vi "MosbusResponseSubVI.vi"(0 "Read String":string) -> (1 "Function Code":i32, 2 "Byte Count":i32, 3 "Data":dbl)   [LabVIEW 2016]
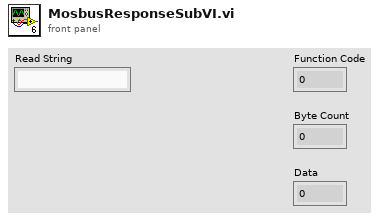
[diagram p1: front panel]
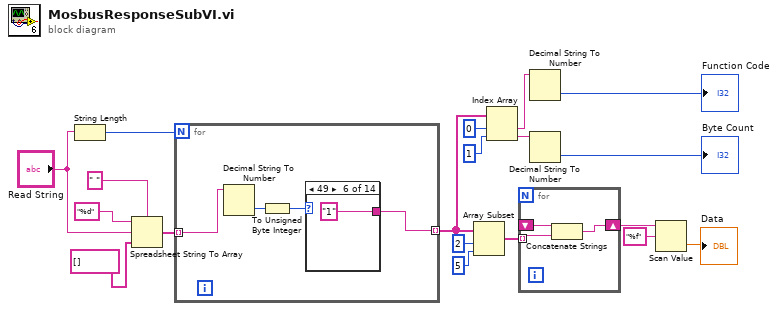
[diagram p0: block diagram]
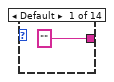
[diagram p2: hidden frame]
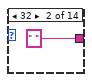
[diagram p3: hidden frame]
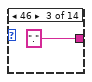
[diagram p4: hidden frame]
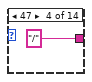
[diagram p5: hidden frame]
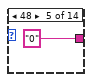
[diagram p6: hidden frame]
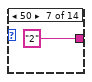
[diagram p7: hidden frame]
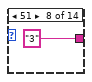
[diagram p8: hidden frame]
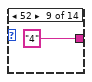
[diagram p9: hidden frame]
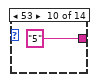
[diagram p10: hidden frame]
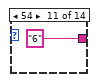
[diagram p11: hidden frame]
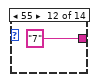
[diagram p12: hidden frame]
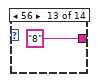
[diagram p13: hidden frame]
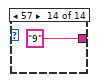
[diagram p14: hidden frame]
diagram:
  n1 = String Length(string="Read String") -> (length=w19:i32)
  n2 = Spreadsheet String To Array(delimiter (Tab)=" ", format string="%d", spreadsheet string="Read String", array type (2D Dbl)=string[] []) -> (array=w4:string[])
  n3 = for {
    N: w19 -> [_]
    tunnel: w4 -> [w20] mode=indexing
    tunnel: [w21] -> w11 mode=indexing
    n4 = Decimal String To Number(string=w20) -> (number=w22:i32)  [unwired: 2 in, 1 out]
    n5 = To Unsigned Byte Integer(number=w22) -> (unsigned 8bit integer=w23:u8)
    n6 = case shown="49" w23 {
      tunnel: ["" " " "." "/" "0" "1" "2" "3" "4" "5" "6" "7" "8" "9"] -> w21
      frame Default {
      }
      frame 32 {
      }
      frame 46 {
      }
      frame 47 {
      }
      frame 48 {
      }
      frame 49 {
      }
      frame 50 {
      }
      frame 51 {
      }
      frame 52 {
      }
      frame 53 {
      }
      frame 54 {
      }
      frame 55 {
      }
      frame 56 {
      }
      frame 57 {
      }
    }
  }
  n7 = Array Subset(array=w11, index=2, length=5) -> (w14:string[])
  n8 = Index Array(array=w11, index #1=0 ("index"), index #2=1 ("index")) -> (element #1=w9:string, element #2=w10:string)
  n9 = for {
    tunnel: w14 -> [w38] mode=indexing
    shift-right: [w40] -> w15
    shift-left: _ -> [w39]
    n10 = Concatenate Strings(w39, w38) -> (w40:string)
  }
  n11 = Decimal String To Number(string=w9) -> (number=→"Function Code":i32)  [unwired: 2 in, 1 out]
  n12 = Decimal String To Number(string=w10) -> (number=→"Byte Count":i32)  [unwired: 2 in, 1 out]
  n13 = Scan Value(string=w15, format string="%f") -> (value=→"Data":dbl)  [unwired: 1 in, 1 out]
